vi "OutdentItem__slk_tc.vi"(0 "tree control in":refnum<class "TreeControl.lvclass">, 5 "outdent tag (current tag)":string, 11 "error in (no error)":errorcluster) -> (4 "tree control out":refnum<class "TreeControl.lvclass">, 15 "error out":errorcluster)   [LabVIEW 2020, in "TreeControl.lvclass"]
doc: "Outdents the currently selected item or the input tag to the same indent level of its parent. Places in the topmost position of its siblings thus disrupting the order. If already at the most mature level in the tree, it moves it to the top of the structure."
uses:
  Library/TreeControl.lvclass
  Library/TreeControl.lvclass/TreeControl.ctl
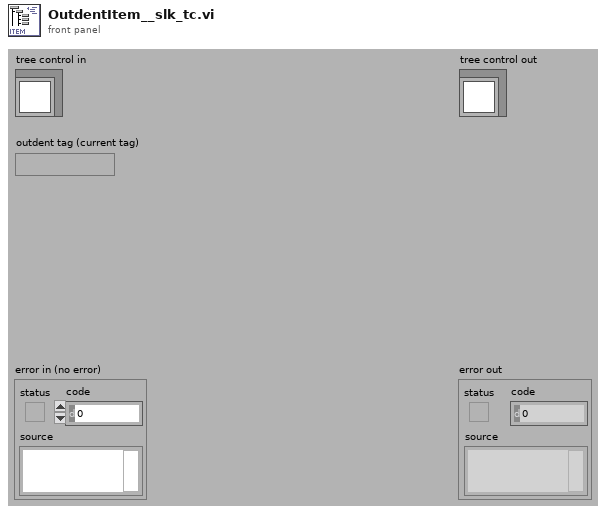
[diagram p1: front panel]
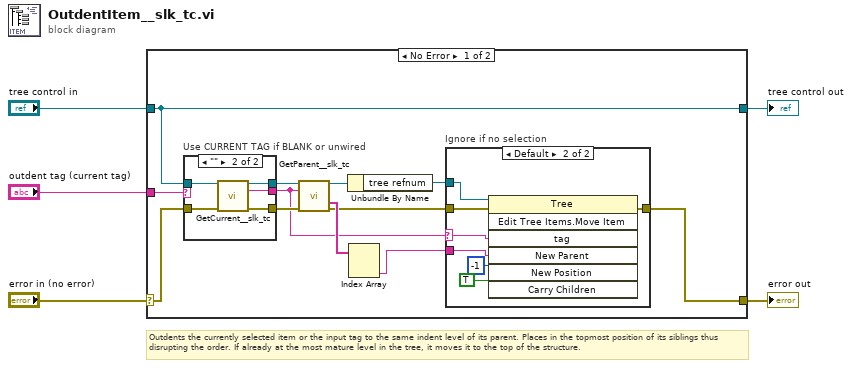
[diagram p0: block diagram]
diagram:
  # "Outdents the currently selected item or the input tag to the same indent level of its parent. Places in the topmost position of its siblings thus disrupting the order. If already at the most mature level in the tree, it moves it to the top of the structure."
  n1 = case shown="No Error" "error in (no error)" {
    selector: "error in (no error)" -> [w7 w35]
    tunnel: [w6 w35] -> w4
    tunnel: [w16 w34] -> w2
    tunnel: "tree control in" -> [w16 w34]
    tunnel: "outdent tag (current tag)" -> [w17 _]
    frame No Error {
      n2 = case "Use CURRENT TAG if BLANK or unwired" shown="\"\"" w17 {
        selector: w17 -> [w28 _]
        tunnel: [w28 w33] -> w12
        tunnel: w16 -> [w26 w32]
        tunnel: w7 -> [w27 w31]
        tunnel: [w27 w30] -> w15
        tunnel: [w26 w29] -> w13
        frame Default {
        }
        frame "" {
          n3 = call "GetCurrent__slk_tc.vi"("tree control in"=w32, "error in (no error)"=w31) -> ("tree control out"=w29:refnum<class "TreeControl.lvclass">, "current tag"=w33:string, "error out"=w30:errorcluster)  [unwired: 1 in, 10 out]
        }
      }
      n4 = call "GetParent__slk_tc.vi"("tree control in"=w13, "child tag (\"\")"=w12, "error in (no error)"=w15) -> ("tree control out"=w11:refnum<class "TreeControl.lvclass">, "parents tags"=w14:string[], "error out"=w9:errorcluster)  [unwired: 10 out]
      n5 = Unbundle By Name(w11) -> ("tree refnum"=w10:refnum<vi>)
      n6 = Index Array(array=w14) -> (element #2=w8:string)  [unwired: 2 in, 1 out]
      n7 = case "Ignore if no selection" shown="Default" w12 {
        selector: w12 -> [_ w23]
        tunnel: w10 -> [_ w25]
        tunnel: w9 -> [w18 w24]
        tunnel: [w18 w21] -> w6
        tunnel: w8 -> [_ w20]
        frame "" {
        }
        frame Default {
          n8 = invoke class="Tree" method="Edit Tree Items.Move Item"(reference=w25, error in=w24, "tag"=w23, "New Parent"=w20, "New Position"=-1, "Carry Children"=TRUE ("Carry Children?")) -> (error out=w21:errorcluster)  [unwired: 1 in, 6 out]
        }
      }
    }
    frame Error {
    }
  }
  "error out" <- w4
  "tree control out" <- w2
